vi "Read Caption.vi"(8 "error in":errorcluster, 11 "Control Reference in":refnum<vi>) -> (0 "error out":errorcluster, 1 "Value":string, 2 "Interpret As Unicode":bool, 3 "Control Reference out":refnum<vi>)   [LabVIEW 2020, in "G-Unicode.lvlib"]
uses:
  G-Unicode.lvlib
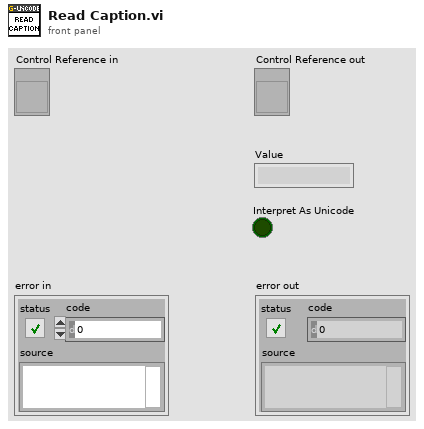
[diagram p1: front panel]
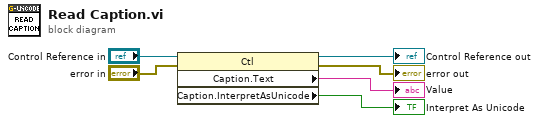
[diagram p0: block diagram]
diagram:
  n1 = property class="Ctl"(reference="Control Reference in", error in="error in") -> (reference out=→"Control Reference out":refnum<vi>, error out=→"error out":errorcluster, "Caption.Text"=→"Value":string, "Caption.InterpretAsUnicode"=→"Interpret As Unicode":bool)
